vi "test_fft2.vi"() -> ()   [LabVIEW 2009]
doc: "Copyright (c) 2010 Stepan A. Baranov (stepan@baranov.su)\nAll rights reserved.\nweb-site: www.OCTLab.org"
uses:
  <vilib>/Analysis/4window.llb/Hanning Window (DBL).vi
  <vilib>/Analysis/NI_AALPro.lvlib
  OCTLib_64.dll
panel:
  out "error out":errorcluster
  out "Im part":dbl[](array[numeric])
  out "Re part":dbl[](array[numeric])
  out "Phase A-scan":dbl[](array[numeric])
  out "Intensity A-scan":dbl[](array[numeric])
  out "Im":dbl[](array[numeric])
  out "Re":dbl[](array[numeric])
  out "phase":dbl[](array[numeric])
  out "intensity":dbl[](array[numeric])
  out "time for FFT":u32
  in  "RSM_STAT?":bool=TRUE
  in  "stop":bool
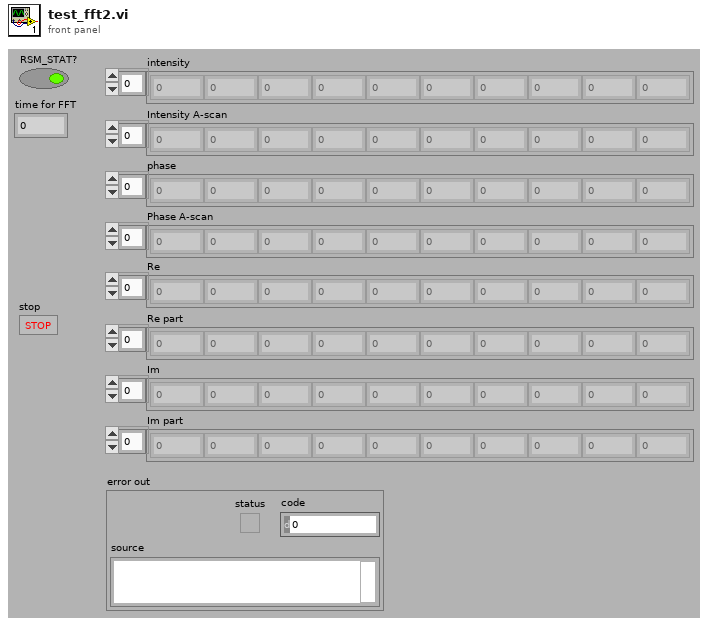
[diagram p1: front panel]
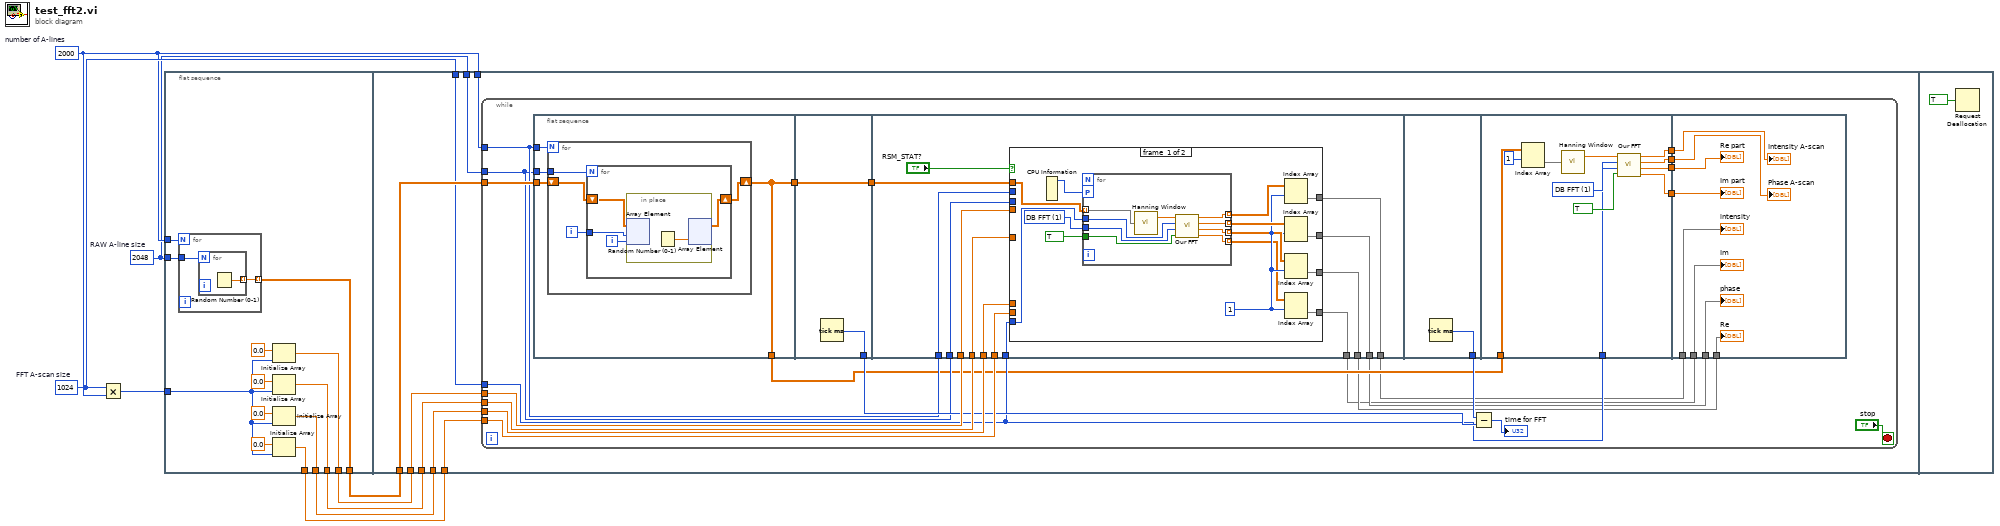
[diagram p0: block diagram]
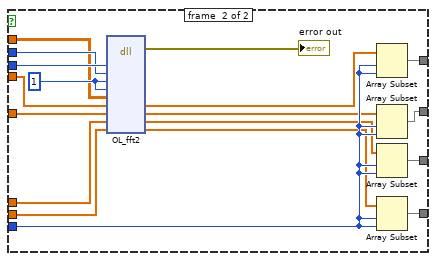
[diagram p2: hidden frame]
diagram:
  w3 = 1024  # FFT A-scan size
  w2 = 2000  # number of A-lines
  w1 = 2048  # RAW A-line size
  n1 = Multiply(x=w3, y=w2) -> (x*y=w9:i32)
  n2 = flat-sequence {
    tunnel: w1 -> [w21]
    tunnel: w2 -> [w20]
    tunnel: w9 -> [w15]
    tunnel: [w14] -> w8
    tunnel: [w13] -> w7
    tunnel: [w12] -> w6
    tunnel: [w11] -> w5
    tunnel: [w10] -> w4
    tunnel: w2 -> [w32]
    tunnel: w1 -> [w31]
    tunnel: w8 -> [w30]
    tunnel: w7 -> [w29]
    tunnel: w6 -> [w28]
    tunnel: w5 -> [w27]
    tunnel: w4 -> [w26]
    tunnel: w3 -> [w25]
    frame #0 {
      n3 = for {
        N: w20 -> [_]
        tunnel: [w23] -> w10 mode=indexing
        tunnel: w21 -> [w22]
        n4 = for {
          N: w22 -> [_]
          tunnel: [w24] -> w23 mode=indexing
          n5 = Random Number (0-1)() -> (number: 0 to 1=w24:dbl)
        }
      }
      n6 = Initialize Array(0.0 ("element"), w15) -> (w13:dbl[])
      n7 = Initialize Array(0.0 ("element"), w15) -> (w12:dbl[])
      n8 = Initialize Array(0.0 ("element"), w15) -> (w14:dbl[])
      n9 = Initialize Array(0.0 ("element"), w15) -> (w11:dbl[])
    }
    frame #1 {
      n10 = while {
        tunnel: w26 -> [w54]
        tunnel: w32 -> [w46]
        tunnel: w31 -> [w45]
        tunnel: w30 -> [w53]
        tunnel: w29 -> [w52]
        tunnel: w28 -> [w51]
        tunnel: w27 -> [w50]
        tunnel: w25 -> [w44]
        stop <- "stop" stop-if-true
        n11 = flat-sequence {
          tunnel: w54 -> [w59]
          tunnel: w46 -> [w58]
          tunnel: w45 -> [w57]
          tunnel: [w56] -> w43
          tunnel: [w56] -> w33
          tunnel: [w70] -> w49
          tunnel: [w69] -> w34
          tunnel: w33 -> [w69]
          tunnel: w53 -> [w82]
          tunnel: w52 -> [w81]
          tunnel: w51 -> [w80]
          tunnel: w50 -> [w79]
          tunnel: w45 -> [w78]
          tunnel: w46 -> [w77]
          tunnel: [w76] -> w38
          tunnel: [w75] -> w37
          tunnel: [w74] -> w36
          tunnel: [w73] -> w35
          tunnel: w44 -> [w72]
          tunnel: w34 -> [w71]
          tunnel: [w125] -> w47
          tunnel: w43 -> [w136]
          tunnel: w44 -> [w130]
          tunnel: [w129] -> w42
          tunnel: [w128] -> w41
          tunnel: [w127] -> w40
          tunnel: [w126] -> w39
          tunnel: w42 -> [w144]
          tunnel: w41 -> [w143]
          tunnel: w40 -> [w142]
          tunnel: w39 -> [w141]
          tunnel: w38 -> [w140]
          tunnel: w37 -> [w139]
          tunnel: w36 -> [w138]
          tunnel: w35 -> [w137]
          frame #0 {
            n12 = for {
              N: w58 -> [_]
              shift-right: [w61] -> w56
              shift-left: w59 -> [w62]
              tunnel: w57 -> [w63]
              i -> [w60]
              n13 = for {
                N: w63 -> [_]
                shift-right: [w64] -> w61
                shift-left: w62 -> [w67]
                tunnel: w60 -> [w66]
                i -> [w65]
                n14 = in-place {
                  n15 = in-place-array #1(w67, w66, w65) -> ()  [unwired: 1 out]
                  n16 = Random Number (0-1)() -> (number: 0 to 1=w68:dbl)
                  n17 = in-place-array #1(w68) -> (w64:dbl[][])  [unwired: 2 out]
                }
              }
            }
          }
          frame #1 {
            n18 = Tick Count (ms)() -> (millisecond timer value=w70:u32)
          }
          frame #2 {
            n19 = case shown="True" "RSM_STAT?" {
              tunnel: w82 -> [_ w121]
              tunnel: w81 -> [_ w124]
              tunnel: w80 -> [_ w123]
              tunnel: w79 -> [_ w122]
              tunnel: w78 -> [_ w120]
              tunnel: w77 -> [_ w119]
              tunnel: w71 -> [w97 w117]
              tunnel: [w94 w115] -> w76
              tunnel: [w92 w112] -> w75
              tunnel: [w91 w110] -> w74
              tunnel: [w88 w108] -> w73
              tunnel: w72 -> [w96 w116]
              frame #0 {
                w84 = 1 items=["LINEAR FFT", "DB FFT"] ("A-scan type")
                w89 = 1 ("index (row)")
                n20 = CPU Information() -> (4:w86:i32)  [unwired: 3 out]
                n21 = for {
                  workers-P: w86 -> [_]
                  tunnel: [w105] -> w95 mode=indexing
                  tunnel: [w104] -> w93 mode=indexing
                  tunnel: [w103] -> w90 mode=indexing
                  tunnel: [w102] -> w87 mode=indexing
                  tunnel: w97 -> [w101] mode=indexing
                  tunnel: w96 -> [w100]
                  tunnel: TRUE ("need phase?") -> [w99]
                  tunnel: w84 -> [w98]
                  n22 = call-poly <vilib>:"Hanning Window.vi"("X"=w101) -> ("Windowed X"=w106:dbl[])  [unwired: 1 out]
                  n23 = call "Our FFT.vi"("need phase?"=w99, "A-scan type"=w98, "FFT A-scan size"=w100, "RAW A-line"=w106) -> ("Im part"=w102:dbl[], "Re part"=w103:dbl[], "Phase A-scan"=w104:dbl[], "Intensity A-scan"=w105:dbl[])
                }
                n24 = Index Array(array=w95, index (row)=w89) -> (element=w94:dbl[])  [unwired: 1 in]
                n25 = Index Array(array=w93, index (row)=w89) -> (element=w92:dbl[])  [unwired: 1 in]
                n26 = Index Array(array=w90, index (row)=w89) -> (element=w91:dbl[])  [unwired: 1 in]
                n27 = Index Array(array=w87, index (row)=w89) -> (element=w88:dbl[])  [unwired: 1 in]
              }
              frame #1 {
                w118 = i8 1 ("hanning_flag")
                n28 = dll-call lib="OCTLib**.*" fn="OL_fft2"("width"=w120, "height"=w119, "hanning_flag"=w118, "log10_flag"=w118, "input"=w117, "intensity"=w124, "phase"=w123, "Re"=w121, "Im"=w122) -> (error out=→"error out":errorcluster, "intensity"=w114:dbl[], "phase"=w113:dbl[], "Re"=w111:dbl[], "Im"=w109:dbl[])  [unwired: 9 in, 1 out]
                n29 = Array Subset(array=w114, index=w116, length=w116) -> (w115:dbl[])
                n30 = Array Subset(array=w113, index=w116, length=w116) -> (w112:dbl[])
                n31 = Array Subset(array=w111, index=w116, length=w116) -> (w110:dbl[])
                n32 = Array Subset(array=w109, index=w116, length=w116) -> (w108:dbl[])
              }
            }
          }
          frame #3 {
            n33 = Tick Count (ms)() -> (millisecond timer value=w125:u32)
          }
          frame #4 {
            w133 = 1 items=["LINEAR FFT", "DB FFT"] ("A-scan type")
            n34 = Index Array(array=w136, index (row)=1) -> (element=w131:dbl[])  [unwired: 1 in]
            n35 = call-poly <vilib>:"Hanning Window.vi"("X"=w131) -> ("Windowed X"=w134:dbl[])  [unwired: 1 out]
            n36 = call "Our FFT.vi"("need phase?"=TRUE, "A-scan type"=w133, "FFT A-scan size"=w130, "RAW A-line"=w134) -> ("Im part"=w126:dbl[], "Re part"=w127:dbl[], "Phase A-scan"=w128:dbl[], "Intensity A-scan"=w129:dbl[])
          }
          frame #5 {
            "Intensity A-scan" <- w144
            "Phase A-scan" <- w143
            "Re part" <- w142
            "Im part" <- w141
            "intensity" <- w140
            "phase" <- w139
            "Re" <- w138
            "Im" <- w137
          }
        }
        n37 = Subtract(x=w47, y=w49) -> (x-y=→"time for FFT":u32)
      }
    }
    frame #2 {
      n38 = Request Deallocation(TRUE ("flag")) -> ()
    }
  }
